vi "Random.vi"(0 "Grids in":i32[][](array[numeric])) -> (1 "Grids out":i32[][](array[numeric]), 2 "Failed?":bool)   [LabVIEW 2018]
doc: "Add random 2 or 4 on Grids."
panel:
  in  "Positions that contains 0":cluster{"i":i32, "j":i32}[](array[cluster])
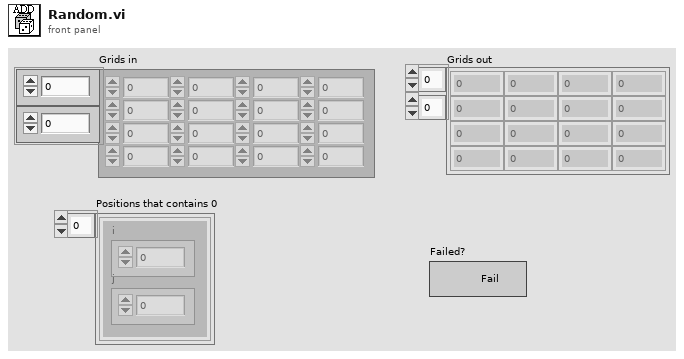
[diagram p1: front panel]
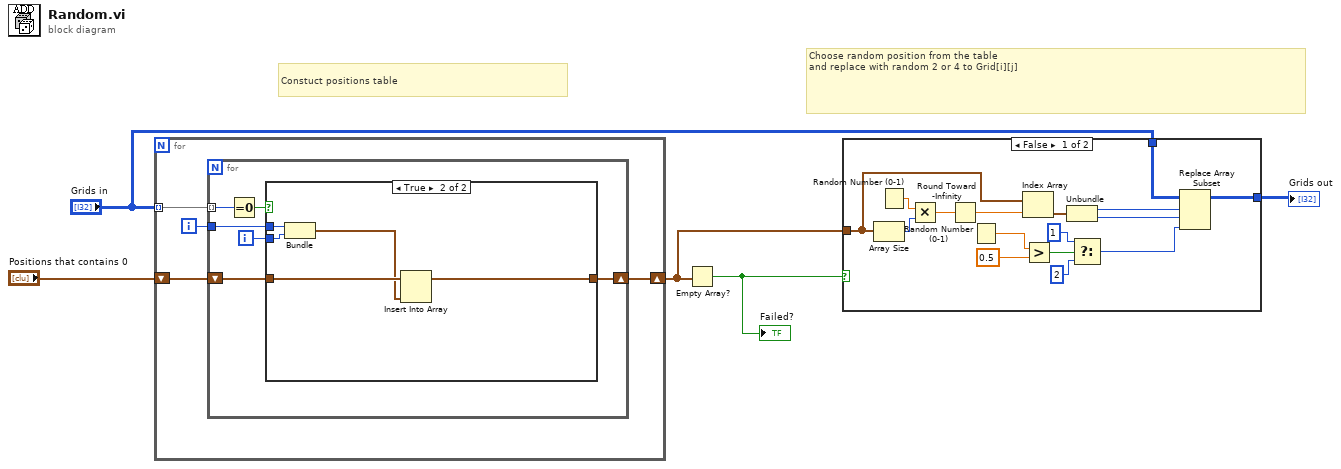
[diagram p0: block diagram]
diagram:
  # "Choose random position from the table \nand replace with random 2 or 4 to Grid[i][j]"
  # "Constuct positions table"
  n1 = for {
    tunnel: "Grids in" -> [w9] mode=indexing
    shift-right: [w6] -> w4
    shift-left: "Positions that contains 0" -> [w7]
    i -> [w8]
    n2 = for {
      tunnel: w9 -> [w15] mode=indexing
      tunnel: w8 -> [w13]
      shift-right: [w10] -> w6
      shift-left: w7 -> [w11]
      i -> [w12]
      n3 = Equal To 0?(x=w15) -> (x = 0?=w14:bool)
      n4 = case shown="True" w14 {
        tunnel: w13 -> [_ w21]
        tunnel: w12 -> [_ w20]
        tunnel: w11 -> [w16 w19]
        tunnel: [w16 w17] -> w10
        frame False {
        }
        frame True {
          n5 = Bundle(w21, w20) -> (w18:cluster{i32, i32})  [unwired: 1 in]
          n6 = Insert Into Array(array=w19, new element=w18) -> (w17:cluster{"i":i32, "j":i32}[])  [unwired: 1 in]
        }
      }
    }
  }
  n7 = Empty Array?(array=w4) -> (empty?=w1:bool)
  "Failed?" <- w1
  n8 = case shown="False" w1 {
    tunnel: w4 -> [w33 _]
    tunnel: "Grids in" -> [w31 w38]
    tunnel: [w28 w38] -> w2
    frame False {
      n9 = Array Size(array=w33) -> (size(s)=w36:i32)
      n10 = Random Number (0-1)() -> (number: 0 to 1=w37:dbl)
      n11 = Multiply(x=w37, y=w36) -> (x*y=w35:dbl)
      n12 = Round Toward -Infinity(1:w35) -> (0:w34:dbl)
      n13 = Random Number (0-1)() -> (number: 0 to 1=w27:dbl)
      n14 = Index Array(array=w33, index=w34) -> (element=w32:cluster{"i":i32, "j":i32})
      n15 = Greater?(x=w27, y=0.5) -> (0:w25:bool)
      n16 = Unbundle(w32) -> ("i"=w30:i32, "j"=w29:i32)
      n17 = Select(t=1, s=w25, f=2) -> (s? t:f=w22:i32)
      n18 = Replace Array Subset(array=w31, new element=w22, index (row)=w30, index (col)=w29) -> (w28:i32[][])
    }
    frame True {
    }
  }
  "Grids out" <- w2
